vi "MGCC_FntStaMach_Watchdog.vi"   [LabVIEW 2016]
doc: "This VI is a watchdog timer. The reset time is set as 10s."
uses:
  <vilib>/RTwatchdog.llb/Watchdog expiration actions.ctl
types:
  T1 = typedef "Watchdog expiration actions.ctl" = cluster{"reset":bool, "occurrence":bool, "trigger protocol":enum16{"active high", "active low", "open collector"}, "trigger line":enum16{"none", "line 0", "line 1", "line 2", "line 3", "line 4", "line 5", "line 6", "line 7", "SMB line 0"}, "disable watchdog on VI exit":bool}
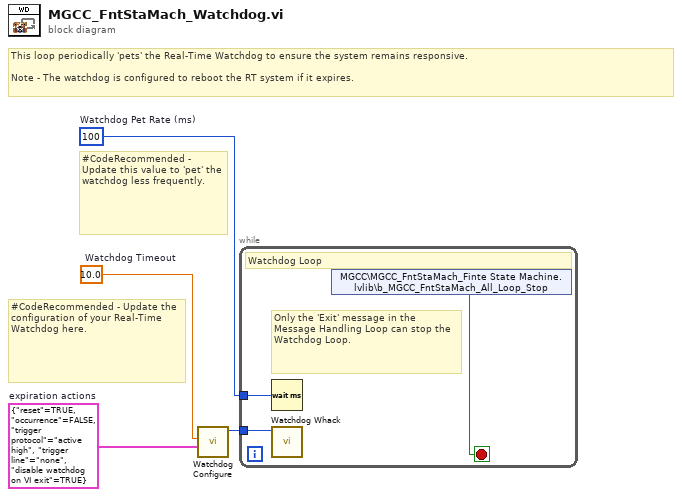
[diagram p0: block diagram]
diagram:
  w1 = u32 100  # Watchdog Pet Rate (ms)
  w2 = T1 {"reset"=TRUE, "occurrence"=FALSE, "trigger protocol"=enum."active high", "trigger line"=enum."none", "disable watchdog on VI exit"=TRUE}  # expiration actions
  w3 = 10.0  # Watchdog Timeout
  # "#CodeRecommended - Update the configuration of your Real-Time Watchdog here."
  # "#CodeRecommended - Update this value to 'pet' the watchdog less frequently."
  # "This loop periodically 'pets' the Real-Time Watchdog to ensure the system remains responsive. \n\nNote - The watchdog is configured to reboot the RT system if it expires."
  n1 = call <vilib>:"Watchdog Configure.vi"("expiration actions"=w2, "timeout (1 sec)"=w3) -> ("watchdogID"=w4:u64)  [unwired: 2 in, 3 out]
  n2 = while {
    tunnel: w4 -> [w6]
    tunnel: w1 -> [w7]
    stop <- w5 stop-if-true
    # "Only the 'Exit' message in the  Message Handling Loop can stop the Watchdog Loop."
    # "Watchdog Loop"
    n3 = Wait (ms)(milliseconds to wait=w7) -> ()  [unwired: 1 out]
    n4 = call <vilib>:"Watchdog Whack.vi"("watchdogID in"=w6) -> ()  [unwired: 4 in, 3 out]
    n5 = shared-variable "MGCC\\MGCC_FntStaMach_Finte State Machine.lvlib\\b_MGCC_FntStaMach_All_Loop_Stop"() -> (w5:bool)  [unwired: 1 in, 1 out]
  }
